vi "libssh2_knownhost_init.vi"(8 "error in (no error)":errorcluster, 11 "session":T1) -> (0 "error out":errorcluster, 3 "known hosts":T2)   [LabVIEW 2013, in "libssh2.lvlib"]
doc: "Initializes a collection of known hosts for this session."
uses:
  libssh2.lvlib
  Known Hosts Refnum.ctl
  Session Refnum.ctl
  libssh2.dll
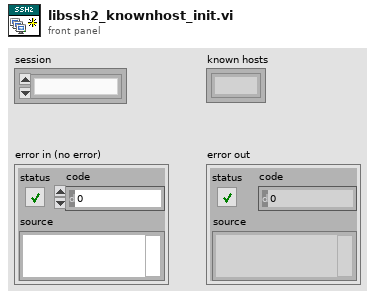
[diagram p1: front panel]
types:
  T1 = typedef "libssh2.lvlib/Session Refnum.ctl" = refnum<k1>
  T2 = typedef "libssh2.lvlib/Known Hosts Refnum.ctl" = refnum<k1>
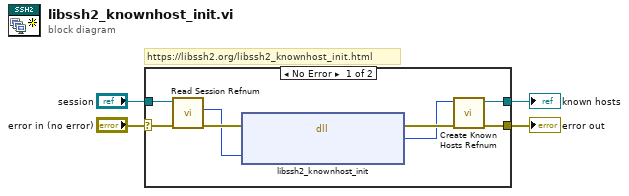
[diagram p0: block diagram]
diagram:
  # "https://libssh2.org/libssh2_knownhost_init.html"
  n1 = case shown="No Error" "error in (no error)" {
    selector: "error in (no error)" -> [w5 w13]
    tunnel: "session" -> [w10 _]
    tunnel: [w8 w13] -> w3
    tunnel: [w6 _] -> w2
    frame No Error {
      n2 = call "Read Session Refnum.vi"("error in (no error)"=w5, "session"=w10) -> ("error out"=w11:errorcluster, "LIBSSH2_SESSION*"=w9:u64)  [unwired: 8 in]
      n3 = dll-call lib="C:/Users/pasca/source/repos/libssh2-labview/libssh2**.*" fn="libssh2_knownhost_init"(error in=w11, "session"=w9) -> (error out=w12:errorcluster, "return value"=w7:u64)  [unwired: 3 in, 1 out]
      n4 = call "Create Known Hosts Refnum.vi"("error in (no error)"=w12, "LIBSSH2_KNOWNHOSTS*"=w7) -> ("error out"=w8:errorcluster, "known hosts"=w6:T2)  [unwired: 8 in]
    }
    frame Error {
    }
  }
  "known hosts" <- w2
  "error out" <- w3
